vi "SetWavelength.vi"(8 "error in (no error)":errorcluster, 10 "Wavelength":dbl, 11 "Device Index":u8) -> (0 "error out":errorcluster, 3 "Device Index":u8)   [LabVIEW 2019, in "TopasDriver.lvlib"]
uses:
  TopasDriver.lvlib
  FemtoLabControl/Libraries/Topas/TopasAPI.dll
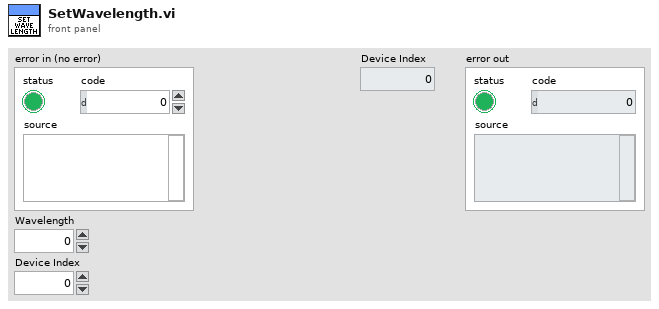
[diagram p1: front panel]
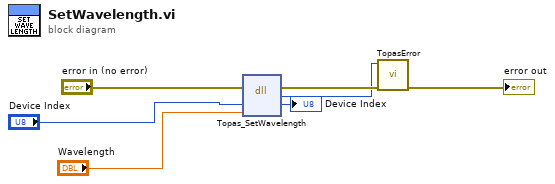
[diagram p0: block diagram]
diagram:
  n1 = dll-call lib="C:/Users/Michael/Documents/GitHub/CampenLab/FemtoLabControl/Libraries/Topas/TopasAPI.dll" fn="Topas_SetWavelength"(error in="error in (no error)", "index"="Device Index", "wl"="Wavelength") -> (error out=w5:errorcluster, "return type"=w3:u32, "index"=→"Device Index":u8)  [unwired: 3 in, 1 out]
  n2 = call "TopasError.vi"("error in"=w5, "Error Code"=w3) -> ("error out"=→"error out":errorcluster)  [unwired: 9 in]
